vi "domeADB_cancelCallback_logEvent_.vi"(8 "error in (no error)":errorcluster) -> (0 "error out":errorcluster, 3 "function return":i32)   [LabVIEW 2015, in "SALLV_domeADB.lvlib"]
doc: "int domeADB_shm_cancelCallback_logeventLV();"
uses:
  SALLV_domeADB.lvlib
  SALLV_domeADB.so
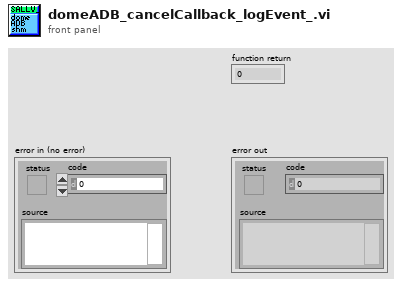
[diagram p1: front panel]
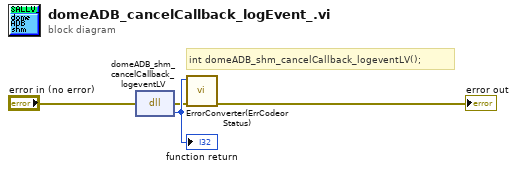
[diagram p0: block diagram]
diagram:
  # "int domeADB_shm_cancelCallback_logeventLV();"
  n1 = dll-call lib="home/andres/Desktop/SALLV_domeADB2015/SALLV_domeADB.*" fn="domeADB_shm_cancelCallback_logeventLV"(error in="error in (no error)") -> (error out=w2:errorcluster, w4:i32)  [unwired: 2 in, 1 out]
  "function return" <- w4
  n2 = call "ErrorConverter(ErrCodeorStatus).vi"("error in (no error)"=w2, "error code"=w4) -> ("error out"=→"error out":errorcluster)  [unwired: 9 in]
